vi "fpga_main_spiral.vi"() -> ()   [LabVIEW 2011]
uses:
  typedefs/DAC_values_cluster.ctl
  typedefs/DAC_voltage_cluster.ctl
  typedefs/cycle_parameters_XY_cluster.ctl
  typedefs/cycle_parameters_cluster.ctl
  typedefs/channels_array.ctl
  typedefs/scan_parameters_cluster.ctl
  typedefs/pixel_to_host_enum.ctl
  typedefs/ramp_parameters_XY_cluster.ctl
  typedefs/ramp_parameters_cluster.ctl
  typedefs/ramp_type_enum.ctl
  typedefs/linear_ramp_parameters_cluster.ctl
  typedefs/sine_ramp_parameters_cluster.ctl
  typedefs/scan_counters_cluster.ctl
  typedefs/cycle_counters_XY_cluster.ctl
  typedefs/cycle_counters_cluster.ctl
  <vilib>/Platform/TimedLoop/XDataNode/timing_clust.ctl
  <vilib>/Platform/TimedLoop/XDataNode/nitl_modes.ctl
  <vilib>/Platform/TimedLoop/XDataNode/wakeup.ctl
  <vilib>/Platform/TimedLoop/XDataNode/XDataNode.xnode
  <vilib>/Platform/TimedLoop/XDataNode/XDNodeRunTimeDep.lvlib
panel:
  in  "Ramp parameters XY":T1
  in  "Bidirectional acquisition":bool
  in  "bitshift":i8
  out "max pixel no.":i64
  in  "pixel-to-host mode":T6=enum."two-channel mode"
  out "Scanning?":bool
  in  "Scan parameters":T7={"No. of waveforms"=11, "Continuous scanning"=TRUE}
  in  "Enable ADC clock?":bool=TRUE
  in  "ADC clock phase":u8
  out "integrated pixel values":T8
  out "data read":T8
  out "FIFO overflow":bool
  out "current pixel no.":i64
  in  "channel offsets":T8
  in  "cycles per pixel":u32=100
  in  "Scan":bool
  in  "wait for trigger?":bool
  in  "stop acquisition at FIFO overflow?":bool
  out "Acquiring?":bool
  in  "Cycle parameters XY":T9={"Cycle parameters X"={"Imaging cycles"=285714, "Settling cycles"=71429, "Resting cycles"=42857, "Phase advance per cycle"=0.0001399517059326172, "Initial Phase"=0.00286865234375}, "Cycle parameters Y"={"Imaging cycles"=285714, "Settling cycles"=71429, "Resting cycles"=42857, "Phase advance per cycle"=0.0001399517059326172, "Initial Phase"=0.00286865234375}}
  out "DAC values to write out":T11 {"bit index" min=-1 max=17 step=1; "channel index" max=7 step=1; "offset" max=4095; "DAC voltage"."ch1" max=4095 step=1; "DAC voltage"."ch0" max=4095 step=1}
  out "In Range?":bool
  in  "Reset DAC":bool
  in  "Stop FPGA":bool
  # "Waveform generation"
  # "Pixel acquisition"
  # "Clock options"
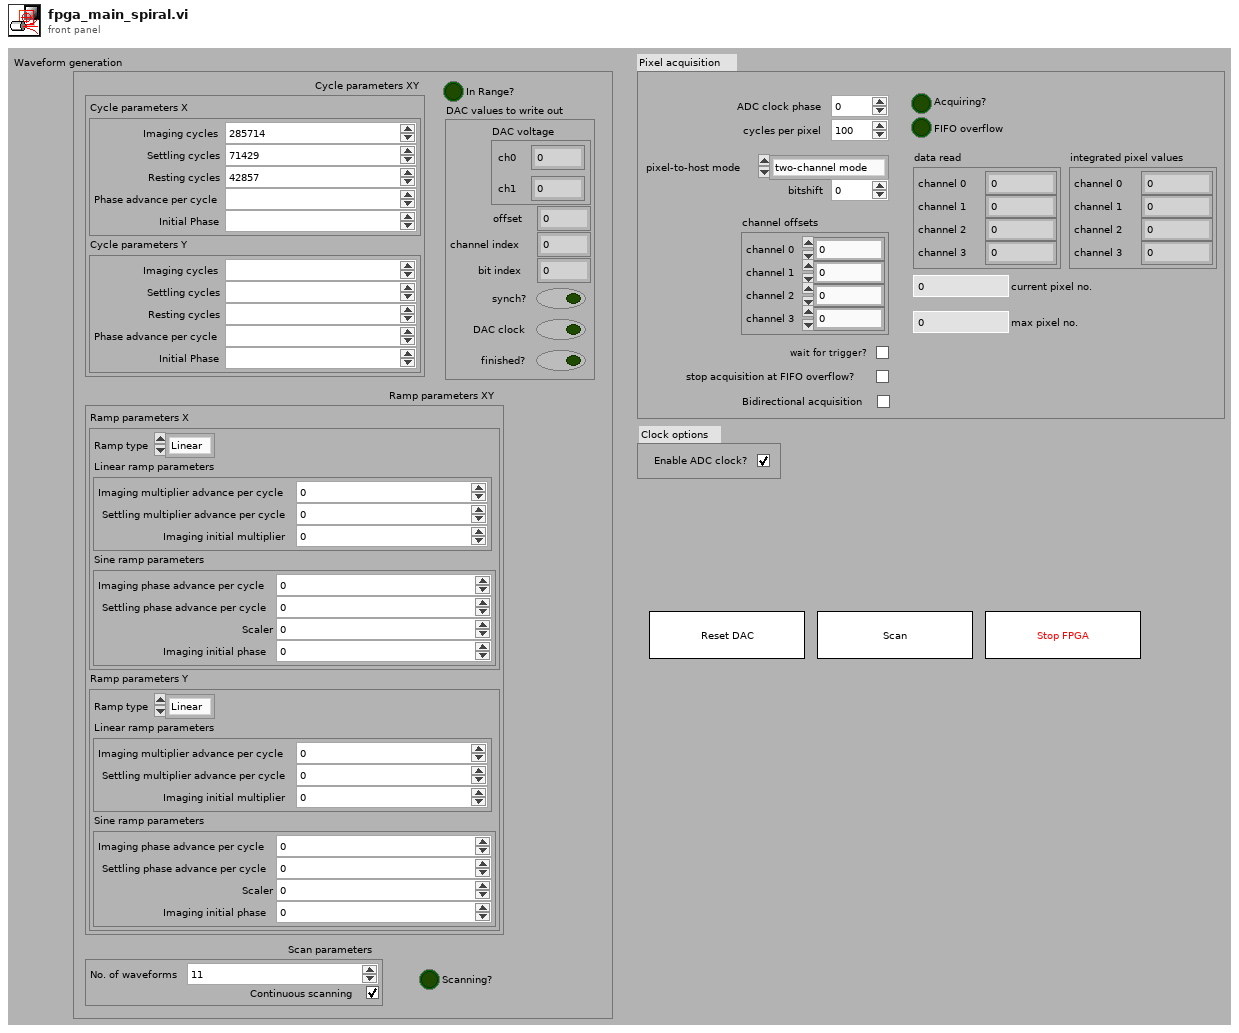
[diagram p1: front panel]
types:
  T1 = typedef "ramp_parameters_XY_cluster.ctl" = cluster{"Ramp parameters X":T2, "Ramp parameters Y":T2}
  T2 = typedef "ramp_parameters_cluster.ctl" = cluster{"Ramp type":T3, "Linear ramp parameters":T4, "Sine ramp parameters":T5}
  T3 = typedef "ramp_type_enum.ctl" = enum8{"Linear", "Sine"}
  T4 = typedef "linear_ramp_parameters_cluster.ctl" = cluster{"Imaging multiplier advance per cycle":fxp<+/-,32,0>, "Settling multiplier advance per cycle":fxp<+/-,32,0>, "Imaging initial multiplier":fxp<+/-,43,12>}
  T5 = typedef "sine_ramp_parameters_cluster.ctl" = cluster{"Imaging phase advance per cycle":fxp<+,32,0>, "Settling phase advance per cycle":fxp<+,32,0>, "Scaler":fxp<+,43,12>, "Imaging initial phase":fxp<+,32,1>}
  T6 = typedef "pixel_to_host_enum.ctl" = enum16{"four-channel mode", "two-channel mode"}
  T7 = typedef "scan_parameters_cluster.ctl" = cluster{"No. of waveforms":u16, "Continuous scanning":bool}
  T8 = typedef "channels_array.ctl" = cluster{"channel 0":u32, "channel 1":u32, "channel 2":u32, "channel 3":u32}
  T9 = typedef "cycle_parameters_XY_cluster.ctl" = cluster{"Cycle parameters X":T10, "Cycle parameters Y":T10}
  T10 = typedef "cycle_parameters_cluster.ctl" = cluster{"Imaging cycles":i32, "Settling cycles":i32, "Resting cycles":i32, "Phase advance per cycle":fxp<+,32,0>, "Initial Phase":fxp<+,32,1>}
  T11 = typedef "DAC_values_cluster.ctl" = cluster{"DAC voltage":T12, "offset":u16, "channel index":u16, "bit index":i32, "synch?":bool, "DAC clock":bool, "finished?":bool}
  T12 = typedef "DAC_voltage_cluster.ctl" = cluster{"ch0":u16, "ch1":u16}
  T13 = typedef "cycle_counters_XY_cluster.ctl" = cluster{"Cycle counters X":T14, "Cycle counters Y":T14}
  T14 = typedef "cycle_counters_cluster.ctl" = cluster{"Imaging counter":i32, "Settling counter":i32, "Resting counter":i32, "Phase":fxp<+,32,1>, "Ramp lin multiplier":fxp<+/-,43,12>, "Ramp sine phase":fxp<+,32,1>}
  T15 = typedef "scan_counters_cluster.ctl" = cluster{"Current part of waveform":u8, "Current waveform":u16}
  T16 = typedef "XDNodeRunTimeDep.lvlib/timing_clust.ctl" = cluster{"Expected End [f-1]":u64, "Actual End [f-1]":u64, "Finished Late? [f-1]":bool, "Expected End [i-1]":u64, "Actual End [i-1]":u64, "Finished Late? [i-1]":bool, "Expected Start [i]":u64, "Actual Start [i]":u64, "Expected Start [f]":u64, "Actual Start [f]":u64, "Source Name":string, "Structure Name":string, "Period":i64, "Deadline":i64, "Offset":i64, "Start":i64, "Priority":i32, "Timeout":i32, "Mode":T17, "Wakeup Reason":T18, "Error":errorcluster, "Source Type":string, "Secondary Source Type":string, "Global End Time":u64, "Global Start Time":u64, "Frame Duration":u64, "Iteration Duration":u64, "Assigned CPU":i32, "I/O Scan Engine Mode":u32}
  T17 = typedef "XDNodeRunTimeDep.lvlib/nitl_modes.ctl" = enum32{"No Change", "Process missed periods, maintain original phase", "Discard missed periods, maintain original phase", "Process missed periods, ignore original phase", "Discard missed periods, ignore original phase"}
  T18 = typedef "XDNodeRunTimeDep.lvlib/wakeup.ctl" = enum32{"Normal", "Aborted", "Asynchronous wakeup", "Timing source error", "Timed loop error", "Timeout"}
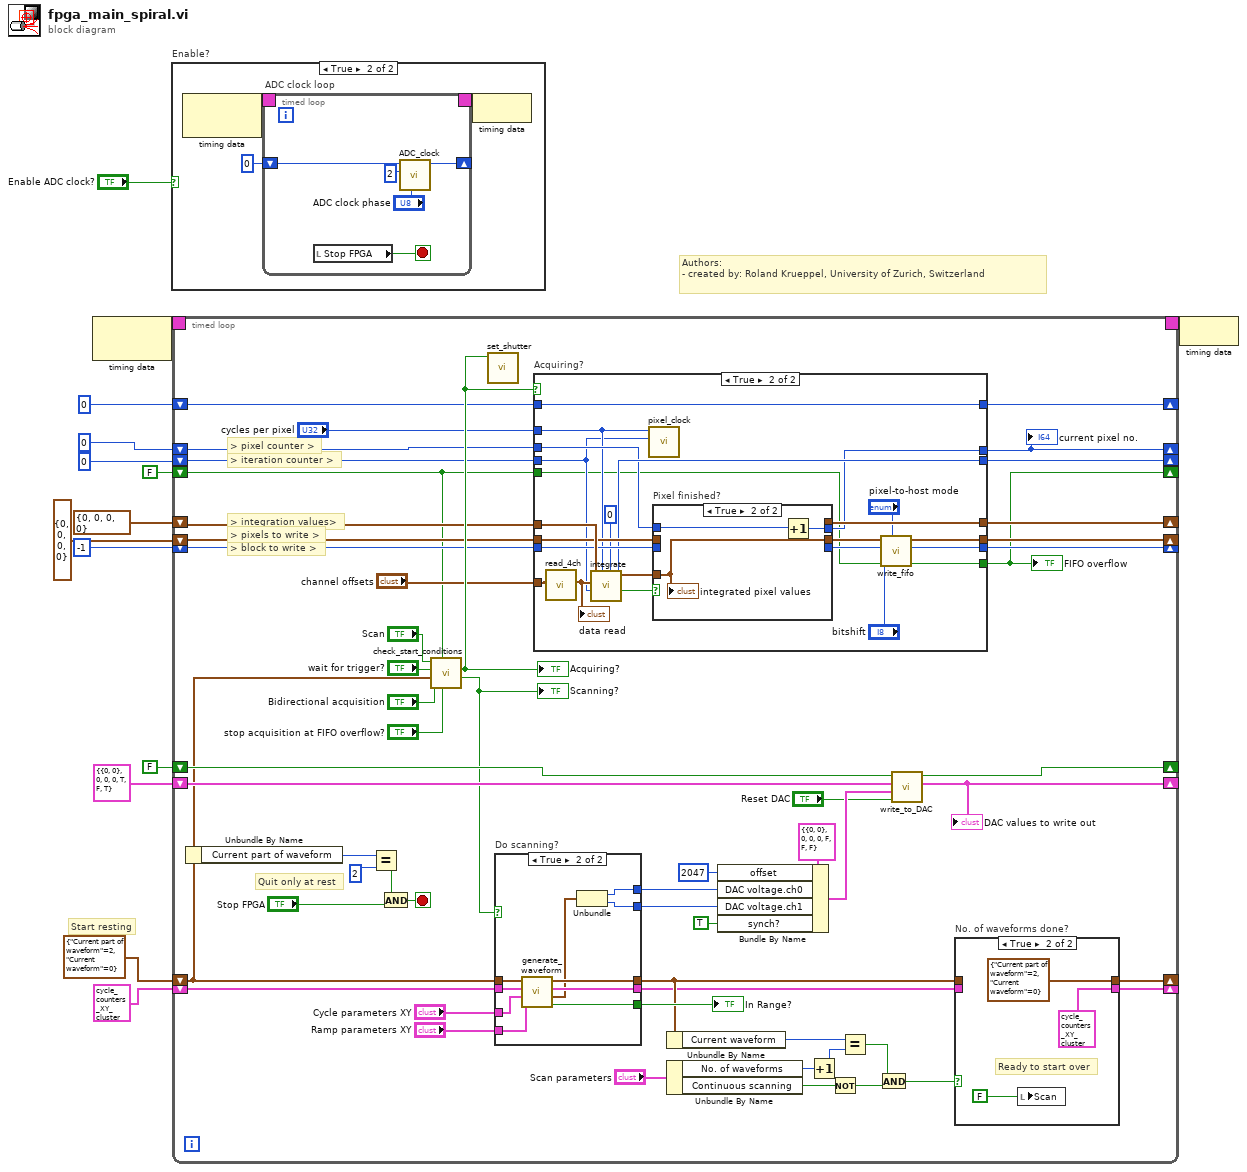
[diagram p0: block diagram]
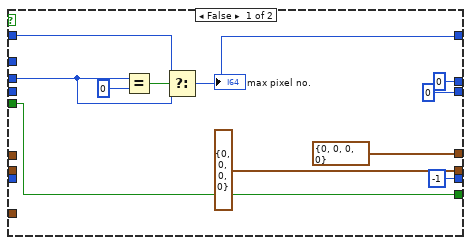
[diagram p3: hidden frame]
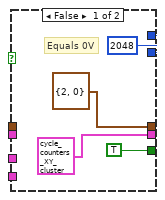
[diagram p6: hidden frame]
diagram:
  # "Authors: \n- created by: Roland Krueppel, University of Zurich, Switzerland"
  # "Start resting"
  n1 = node-c288() -> (w14:T16)  [unwired: 1 in]
  n2 = case "Enable?" shown="True" "Enable ADC clock?" {
    frame False {
    }
    frame True {
      n3 = node-c288() -> (w17:T16)  [unwired: 1 out]
      n4 = timed-loop "ADC clock loop" {
        timing: w17 -> [_]
        timing-out: [_] -> w16
        shift-right: [w21] -> _
        shift-left: u8 0 ("counter out") -> [w22]
        stop <- w18 stop-if-true
        n5 = local read "Stop FPGA"() -> (w18:bool)
        n6 = call "ADC_clock.vi"("phase"="ADC clock phase", "iterations per cycle"=u8 2, "counter in"=w22) -> ("counter out"=w21:u8)  [unwired: 8 in]
      }
      n7 = node-c288(w16) -> ()
    }
  }
  n8 = timed-loop {
    timing: w14 -> [_]
    timing-out: [_] -> w13
    shift-right: [w78] -> _
    shift-left: T11 {"DAC voltage"={"ch0"=0, "ch1"=0}, "offset"=0, "channel index"=0, "bit index"=0, "synch?"=TRUE, "DAC clock"=FALSE, "finished?"=TRUE} ("DAC values to write out") -> [w76]
    shift-right: [w77] -> _
    shift-left: FALSE ("DAC Reset out") -> [w51]
    shift-right: [w30] -> _
    shift-left: T13 {"Cycle counters X"={"Imaging counter"=0, "Settling counter"=0, "Resting counter"=0, "Phase"=0.0, "Ramp lin multiplier"=0.0, "Ramp sine phase"=0.0}, "Cycle counters Y"={"Imaging counter"=0, "Settling counter"=0, "Resting counter"=0, "Phase"=0.0, "Ramp lin multiplier"=0.0, "Ramp sine phase"=0.0}} ("FPGA Cycle Counters XY In") -> [w39]
    shift-right: [w63] -> _
    shift-left: T8 {"channel 0"=0, "channel 1"=0, "channel 2"=0, "channel 3"=0} ("new pixel values out") -> [w62]
    shift-right: [w60] -> _
    shift-left: -1 ("block index out") -> [w58]
    shift-right: [w61] -> _
    shift-left: T8 {"channel 0"=0, "channel 1"=0, "channel 2"=0, "channel 3"=0} ("channels out") -> [w59]
    shift-right: [w55] -> _
    shift-left: FALSE ("FIFO overflow out") -> [w29]
    shift-right: [w56] -> _
    shift-left: u32 0 ("iteration counter out") -> [w53]
    shift-right: [w57] -> _
    shift-left: i64 0 -> [w54]
    shift-right: [w46] -> _
    shift-left: T15 {"Current part of waveform"=2, "Current waveform"=0} ("FPGA Scan Counters In") -> [w36]
    shift-right: [w37] -> _
    shift-left: i64 0 -> [w38]
    stop <- w48 stop-if-true
    # "Quit only at rest"
    # "> pixel counter >"
    # "> block to write >"
    # "> integration values>"
    # "> pixels to write >"
    # "> iteration counter >"
    n9 = Unbundle By Name(w36) -> ("Current part of waveform"=w43:u8)
    n10 = Equal?(x=w43, y=u8 2) -> (x = y?=w41:bool)
    n11 = And(x=w41, y="Stop FPGA") -> (x .and. y?=w48:bool)
    n12 = call "check_start_conditions.vi"("stop at FIFO overflow?"="stop acquisition at FIFO overflow?", "FIFO overflow?"=w29, "Bidirectional acquisition"="Bidirectional acquisition", "FPGA Scan Counters"=w36, "wait for trigger?"="wait for trigger?", "Scan"="Scan") -> ("Scanning?"=w44:bool, "acquire?"=w68:bool)  [unwired: 4 in]
    "Acquiring?" <- w68
    "Scanning?" <- w44
    n13 = call "set_shutter.vi"("open?"=w68) -> ()  [unwired: 11 in]
    n14 = case "Do scanning?" shown="True" w44 {
      tunnel: w39 -> [_ w140]
      tunnel: [w131 w134] -> w75
      tunnel: [w131 w133] -> w74
      tunnel: "Cycle parameters XY" -> [_ w139]
      tunnel: [T13 {"Cycle counters X"={"Imaging counter"=0, "Settling counter"=0, "Resting counter"=0, "Phase"=0.0, "Ramp lin multiplier"=0.0, "Ramp sine phase"=0.0}, "Cycle counters Y"={"Imaging counter"=0, "Settling counter"=0, "Resting counter"=0, "Phase"=0.0, "Ramp lin multiplier"=0.0, "Ramp sine phase"=0.0}} ("FPGA Cycle Counters XY In") w137] -> w31
      tunnel: [TRUE w136] -> w70
      tunnel: w36 -> [_ w141]
      tunnel: [T15 {"Current part of waveform"=2, "Current waveform"=0} ("FPGA Scan Counters In") w138] -> w34
      tunnel: "Ramp parameters XY" -> [_ w132]
      frame False {
        w131 = u16 2048 ("Coerced X")
        # "Equals 0V"
      }
      frame True {
        n15 = call "generate_waveform.vi"("Ramp parameters XY"=w132, "Cycle parameters XY"=w139, "Cycle counters XY In"=w140, "Scan counters in"=w141) -> ("In range"=w136:bool, "Waveform out"=w135:cluster{"Coerced Out":u16, "Coerced Out":u16}, "Cycle counters XY out"=w137:T13, "Scan counters out"=w138:T15)  [unwired: 4 in]
        n16 = Unbundle(w135) -> ("Coerced Out"=w134:u16, "Coerced Out"=w133:u16)
      }
    }
    "In Range?" <- w70
    n17 = case "Acquiring?" shown="True" w68 {
      tunnel: [T8 {"channel 0"=0, "channel 1"=0, "channel 2"=0, "channel 3"=0} ("new pixel values out") w110] -> w63
      tunnel: w62 -> [_ w115]
      tunnel: [T8 {"channel 0"=0, "channel 1"=0, "channel 2"=0, "channel 3"=0} ("channels out") w114] -> w61
      tunnel: w59 -> [_ w107]
      tunnel: [-1 ("block index out") w113] -> w60
      tunnel: w58 -> [_ w109]
      tunnel: w53 -> [_ w98]
      tunnel: [u32 0 ("iteration counter out") w105] -> w56
      tunnel: [w92 w96] -> w55
      tunnel: w54 -> [w82 w103]
      tunnel: [i64 0 w102] -> w57
      tunnel: "channel offsets" -> [_ w100]
      tunnel: "cycles per pixel" -> [_ w99]
      tunnel: w29 -> [w92 w97]
      tunnel: w38 -> [w83 w94]
      tunnel: [w86 w94] -> w37
      frame False {
        n18 = Equal?(x=w82, y=i64 0) -> (x = y?=w84:bool)
        n19 = Select(t=w83, s=w84, f=w82) -> (s? t:f=w86:i64)
        "max pixel no." <- w86
      }
      frame True {
        n20 = call "read_4ch.vi"("channel offsets"=w100) -> ("read output"=w111:T8)  [unwired: 10 in]
        "data read" <- w111
        n21 = call "integrate.vi"("waiting iterations per pixel"=u32 0, "integration iterations per pixel"=w99, "iteration counter in"=w98, "sampling values in"=w111, "previous pixel values in"=w115) -> ("finished?"=w104:bool, "iteration counter out"=w105:u32, "new pixel values out"=w112:T8)  [unwired: 4 in]
        n22 = call "pixel_clock.vi"("current iteration"=w98, "iterations per pixel"=w99) -> ()  [unwired: 10 in]
        n23 = case "Pixel finished?" shown="True" w104 {
          tunnel: w112 -> [w119 w120]
          tunnel: [w119 _] -> w110
          tunnel: w109 -> [w118 _]
          tunnel: [w118 _] -> w108
          tunnel: w107 -> [w117 _]
          tunnel: [w117 w120] -> w106
          tunnel: w103 -> [w116 w122]
          tunnel: [w116 w121] -> w102
          frame False {
          }
          frame True {
            n24 = Increment(x=w122) -> (x+1=w121:i64)
            "integrated pixel values" <- w120
          }
        }
        n25 = call "write_fifo.vi"("pixel-to-host mode"="pixel-to-host mode", "FIFO overflow in"=w97, "bitshift"="bitshift", "block index in"=w108, "values to be written"=w106) -> ("FIFO overflow out"=w96:bool, "block index out"=w113:i32, "channels out"=w114:T8)  [unwired: 4 in]
      }
    }
    "FIFO overflow" <- w55
    "current pixel no." <- w57
    n26 = Unbundle By Name(w34) -> ("Current waveform"=w35:u16)
    n27 = Unbundle By Name("Scan parameters") -> ("No. of waveforms"=w33:u16, "Continuous scanning"=w73:bool)
    n28 = Bundle By Name(cluster=T11 {"DAC voltage"={"ch0"=0, "ch1"=0}, "offset"=0, "channel index"=0, "bit index"=0, "synch?"=FALSE, "DAC clock"=FALSE, "finished?"=FALSE} ("New DAC values generated"), "offset"=u16 2047, "DAC voltage.ch0"=w75, "DAC voltage.ch1"=w74, "synch?"=TRUE) -> (w79:T11)
    n29 = Increment(x=w33) -> (x+1=w32:u16)
    n30 = Not(x=w73) -> (.not. x?=w72:bool)
    n31 = Equal?(x=w35, y=w32) -> (x = y?=w71:bool)
    n32 = And(x=w71, y=w72) -> (x .and. y?=w69:bool)
    n33 = call "write_to_DAC.vi"("DAC New Reset"="Reset DAC", "New DAC values generated"=w79, "DAC values to write In"=w76, "DAC Reset State In"=w51) -> ("DAC values to write out"=w78:T11, "DAC Reset State out"=w77:bool)  [unwired: 3 in]
    "DAC values to write out" <- w78
    n34 = case "No. of waveforms done?" shown="True" w69 {
      tunnel: w34 -> [w124 _]
      tunnel: [w124 T15 {"Current part of waveform"=2, "Current waveform"=0} ("FPGA Scan Counters In")] -> w46
      tunnel: w31 -> [w123 _]
      tunnel: [w123 T13 {"Cycle counters X"={"Imaging counter"=0, "Settling counter"=0, "Resting counter"=0, "Phase"=0.0, "Ramp lin multiplier"=0.0, "Ramp sine phase"=0.0}, "Cycle counters Y"={"Imaging counter"=0, "Settling counter"=0, "Resting counter"=0, "Phase"=0.0, "Ramp lin multiplier"=0.0, "Ramp sine phase"=0.0}} ("FPGA Cycle Counters XY In")] -> w30
      frame False {
      }
      frame True {
        # "Ready to start over"
        n35 = local write "Scan"(FALSE ("Do Scanning")) -> ()
      }
    }
  }
  n36 = node-c288(w13) -> ()
